vi "Set Default Sample Period.vi"(0 "Sample Period (msec)":i32, 1 "Plugin Name":T2, 3 "error in (no error)":errorcluster) -> (4 "Result":T1, 5 "Sample Period (msec) out":i32, 6 "Plugin Name out":T2, 7 "Changed?":bool, 8 "error out":errorcluster)   [LabVIEW 2015, in "Config Data.lvlib" / "Config Data.lvclass"]
uses:
  Config Data.lvclass
  Startup Processes/_typedefs/Subpanel Names.ctl
  Startup Processes/_typedefs/Pass Fail Flag.ctl
  _buffers/Sample Rate/Sample Rate.lvlib
  Startup Processes/Startup Processes.lvlib
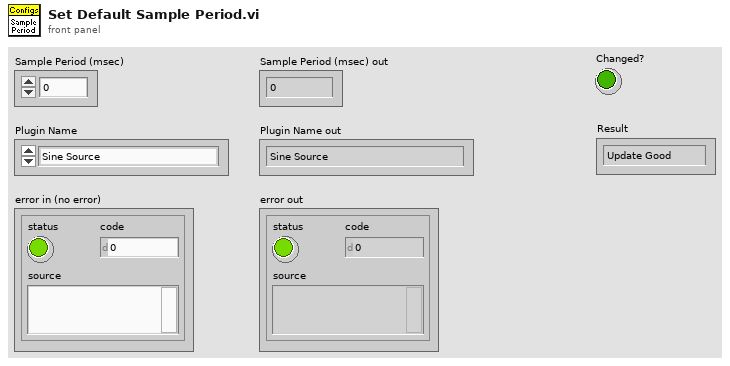
[diagram p1: front panel]
types:
  T1 = typedef "Startup Processes.lvlib/Pass Fail Flag.ctl" = enum16{"Update Good", "Update Failed"}
  T2 = typedef "Startup Processes.lvlib/Subpanel Names.ctl" = enum16{"Sine Source", "Ramp Source", "Hen House TC", "Dog House TC", "Out House TC"}
  T3 = typedef "Startup Processes.lvlib/Data Valid Flag.ctl" = enum16{"Data Valid", "Data Not Valid"}
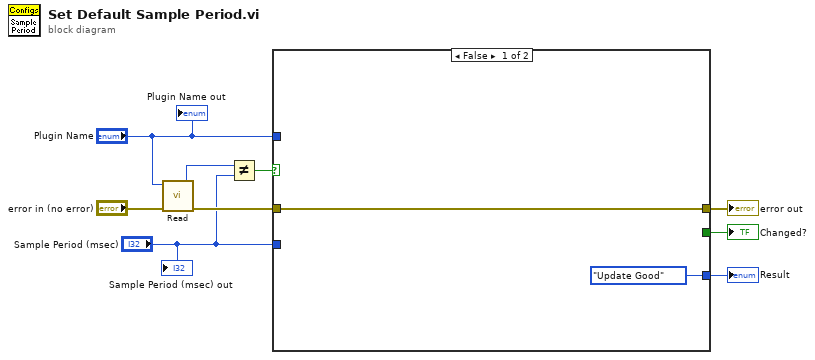
[diagram p0: block diagram]
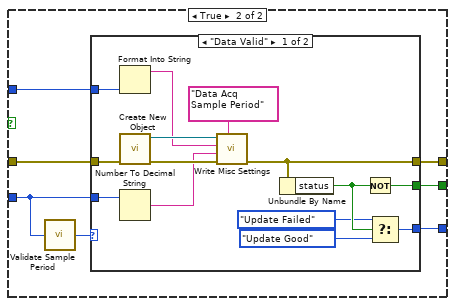
[diagram p2: hidden frame]
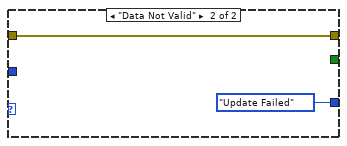
[diagram p3: hidden frame]
diagram:
  n1 = call "Read.vi"("Error In"="error in (no error)", "Plugin Name"="Plugin Name") -> ("Error Out"=w7:errorcluster, "Sample Period (msec)"=w5:i32)  [unwired: 4 in]
  n2 = Not Equal?(x=w5, y="Sample Period (msec)") -> (x != y?=w6:bool)
  n3 = case shown="False" w6 {
    tunnel: [w11 w16] -> w9
    tunnel: "Sample Period (msec)" -> [_ w13]
    tunnel: "Plugin Name" -> [_ w18]
    tunnel: w7 -> [w11 w17]
    tunnel: [_ w15] -> w2
    tunnel: [Pass_Fail_Flag."Update Good" ("Result") w14] -> w1
    frame False {
    }
    frame True {
      n4 = call "Validate Sample Period.vi"("Sample Period (msec)"=w13) -> ("Result"=w12:T3)
      n5 = case shown="\"Data Valid\"" w12 {
        tunnel: w13 -> [w27 _]
        tunnel: w18 -> [w26 _]
        tunnel: w17 -> [w25 w34]
        tunnel: [w24 w34] -> w16
        tunnel: [w23 _] -> w15
        tunnel: [w22 Pass_Fail_Flag."Update Failed" ("Result")] -> w14
        frame "Data Valid" {
          n6 = Format Into String(w26) -> (resulting string=w30:string)  [unwired: 3 in, 1 out]
          n7 = call "Create New Object.vi"("Error In"=w25) -> ("Error Out"=w32:errorcluster, "Config Data"=w31:refnum<class "Config Data.lvclass">)  [unwired: 5 in]
          n8 = Number To Decimal String(number=w27) -> (decimal integer string=w29:string)  [unwired: 1 in]
          n9 = call-dynamic "Write Misc Settings.vi"("Section"="Data Acq Sample Period" ("format string"), "error in (no error)"=w32, "p_value"=w29, "Key"=w30, "Config Data in"=w31) -> ("error out"=w24:errorcluster)  [unwired: 2 in, 1 out]
          n10 = Unbundle By Name(w24) -> ("status"=w21:bool)
          n11 = Not(x=w21) -> (.not. x?=w23:bool)
          n12 = Select(t=Pass_Fail_Flag."Update Failed" ("Result"), s=w21, f=Pass_Fail_Flag."Update Good" ("Result")) -> (s? t:f=w22:T1)
        }
        frame "Data Not Valid" {
        }
      }
    }
  }
  "error out" <- w9
  "Changed?" <- w2
  "Result" <- w1
  "Plugin Name out" <- "Plugin Name"
  "Sample Period (msec) out" <- "Sample Period (msec)"
